vi "detection test.vi"() -> ()   [LabVIEW 2014]
uses:
  <vilib>/Math Plots/3D Math Plots/3D Ribbon/3D Ribbon XCtrl/3D Ribbon.xctl
  <vilib>/Math Plots/2D Math Plots/2D Compass/2D Compass XCtrl/2D Compass.xctl
  <vilib>/Math Plots/3D Math Plots/3D Ribbon/3D Ribbon Datatype/3D Ribbon Datatype.lvclass
  <vilib>/Math Plots/2D Math Plots/2D Compass/2D Compass Datatype/2D Compass Datatype.lvclass
panel:
  out "list":T1(array[cluster])
  in  "Take Reading":bool
  in  "Heading (deg)":dbl(knob)=90.0
  out "2D Compass":refnum<class "2D Plot Datatype.lvclass">[](xcontrol)
  out "Waveform Graph":dbl[][](graph)
  out "3D Ribbon":refnum<class "3D Plot Datatype.lvclass">[](xcontrol)
  in  "Stop":bool
  out "Zone":u8
  out "array":u8[](array[numeric])
  in  "Detectors":T2 {"Det 5" scale=0.0..255.0; "Det 4" scale=0.0..255.0; "Det 3" scale=0.0..255.0; "Det 2" scale=0.0..255.0; "Det 1" scale=0.0..255.0}
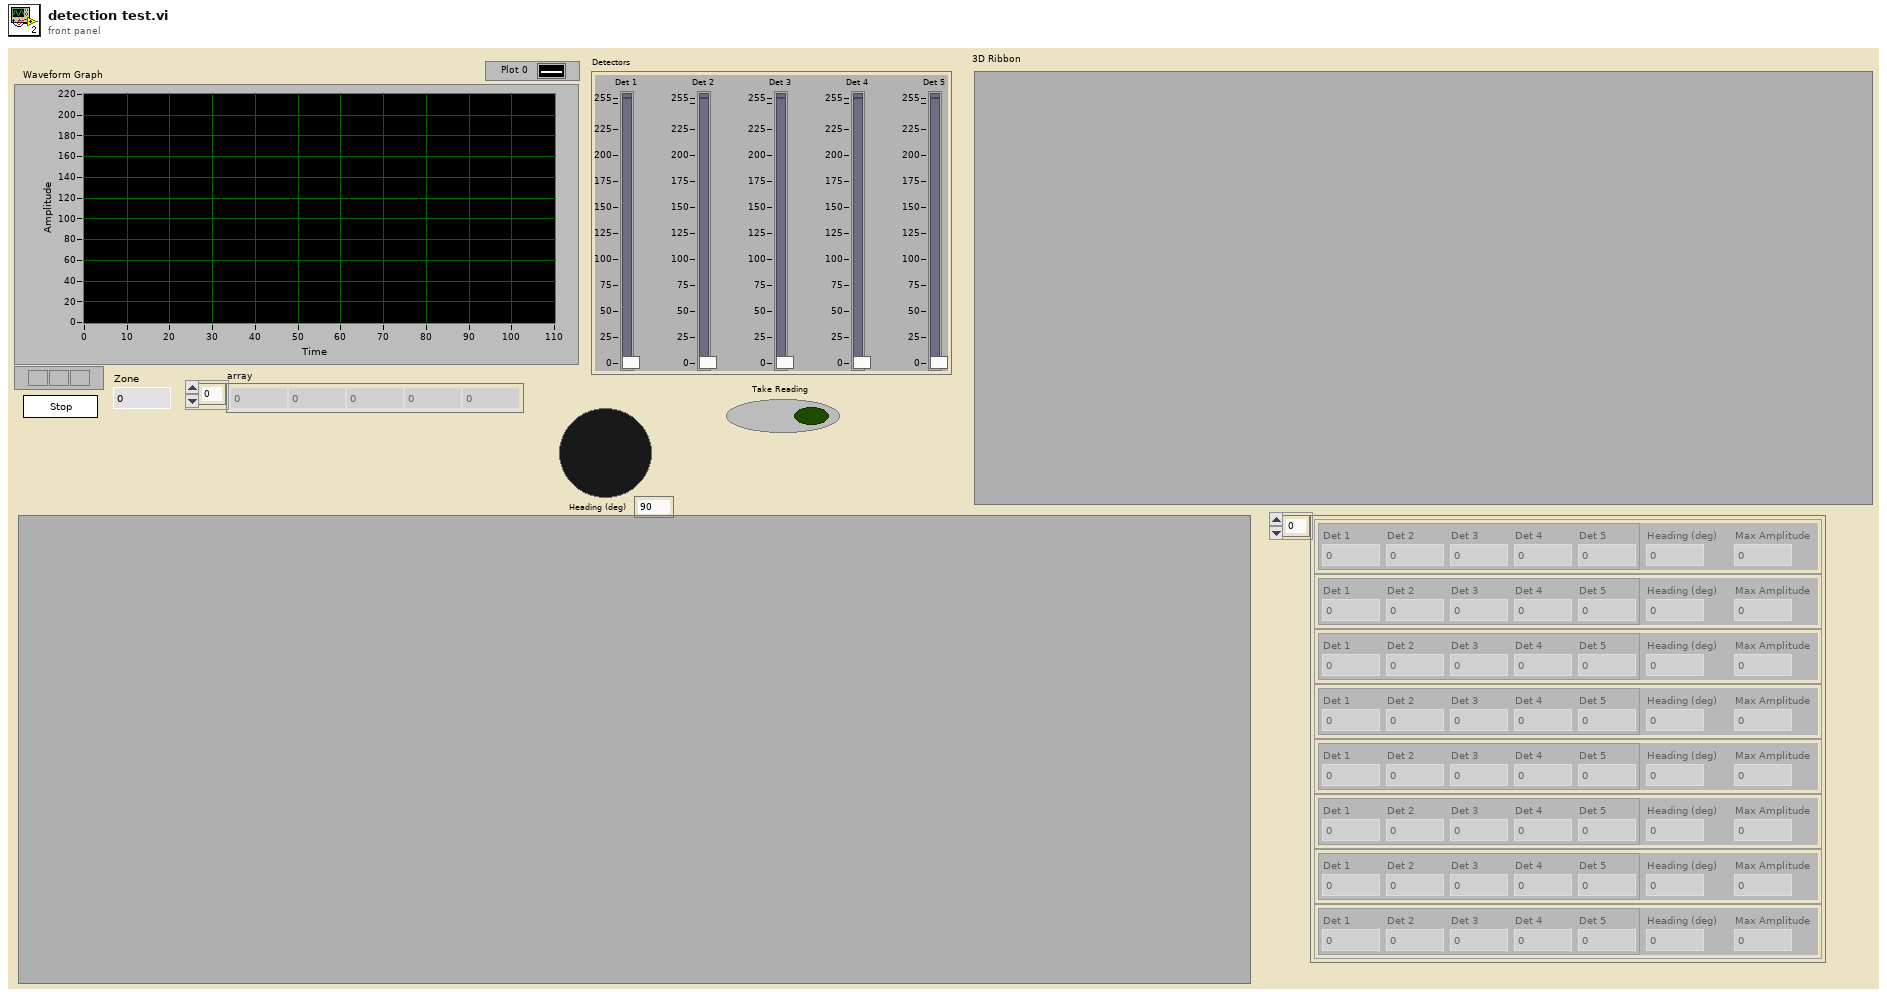
[diagram p1: front panel]
types:
  T1 = cluster{"Detectors":cluster{"Det 1":u8, "Det 2":u8, "Det 3":u8, "Det 4":u8, "Det 5":u8}, "Heading (deg)":dbl, "Max Amplitude":dbl}[]
  T2 = cluster{"Det 1":u8, "Det 2":u8, "Det 3":u8, "Det 4":u8, "Det 5":u8}
  T3 = cluster{"Detectors":cluster{"Det 1":u8, "Det 2":u8, "Det 3":u8, "Det 4":u8, "Det 5":u8}, "Heading (deg)":dbl, "Max Amplitude":dbl}
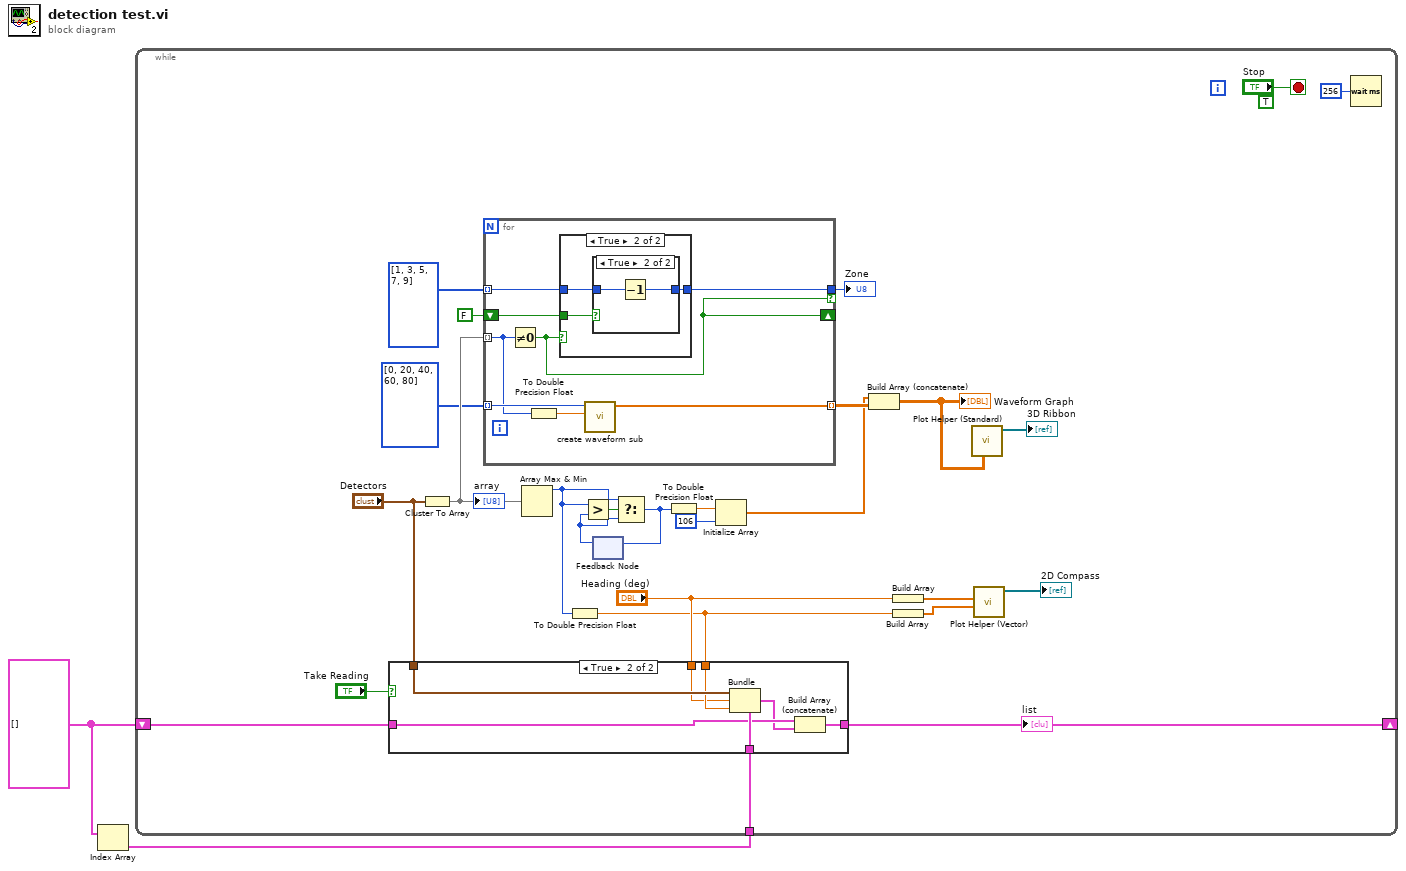
[diagram p0: block diagram]
diagram:
  w2 = T1 [] ("appended array")
  n1 = Index Array(array=w2) -> (element=w1:T3)  [unwired: 1 in]
  n2 = while {
    shift-right: [w10] -> _
    shift-left: w2 -> [w11]
    tunnel: w1 -> [w13]
    stop <- "Stop" stop-if-true
    (unwired) TRUE
    n3 = Cluster To Array(cluster="Detectors") -> (array=w26:u8[])
    "array" <- w26
    n4 = for {
      tunnel: w26 -> [w40] mode=indexing
      shift-right: [w42] -> _
      shift-left: FALSE -> [w45]
      tunnel: u8[] [1, 3, 5, 7, 9] ("array") -> [w44] mode=indexing
      tunnel: [w43] -> w27 if=w42
      tunnel: u8[] [0, 20, 40, 60, 80] ("array") -> [w41] mode=indexing
      tunnel: [w38] -> w20 mode=indexing
      n5 = Not Equal To 0?(x=w40) -> (x != 0?=w42:bool)
      n6 = To Double Precision Float(number=w40) -> (double precision float=w39:dbl)
      n7 = case shown="True" w42 {
        tunnel: w45 -> [_ w49]
        tunnel: w44 -> [w46 w48]
        tunnel: [w46 w47] -> w43
        frame False {
        }
        frame True {
          n8 = case shown="True" w49 {
            tunnel: [w50 w51] -> w47
            tunnel: w48 -> [w50 w52]
            frame False {
            }
            frame True {
              n9 = Decrement(x=w52) -> (x-1=w51:u8)
            }
          }
        }
      }
      n10 = call "create waveform sub.vi"("amplitude"=w39, "index"=w41) -> ("Array"=w38:dbl[])  [unwired: 9 in]
    }
    "Zone" <- w27
    n11 = Array Max & Min(array=w26) -> (max value=w4:u8)  [unwired: 3 out]
    n12 = To Double Precision Float(number=w4) -> (double precision float=w3:dbl)
    n13 = case shown="True" "Take Reading" {
      tunnel: "Detectors" -> [_ w37]
      tunnel: w3 -> [_ w36]
      tunnel: w13 -> [_ w35]
      tunnel: [w30 w34] -> w10
      tunnel: w11 -> [w30 w32]
      tunnel: "Heading (deg)" -> [_ w33]
      frame False {
      }
      frame True {
        n14 = Bundle(cluster=w35, "Detectors"=w37, "Heading (deg)"=w33, "Max Amplitude"=w36) -> (w31:T3)
        n15 = Build Array (concatenate)(w32, w31) -> (w34:T1)
      }
    }
    "list" <- w10
    n16 = feedback #1() -> (w24:u8)  [unwired: 1 in]
    n17 = Greater?(x=w4, y=w24) -> (0:w25:bool)
    n18 = Select(t=w4, s=w25, f=w24) -> (s? t:f=w23:u8)
    n19 = feedback-in #1(w23) -> ()
    n20 = To Double Precision Float(number=w23) -> (double precision float=w6:dbl)
    n21 = Initialize Array(w6, 106 ("dimension size")) -> (w19:dbl[])
    n22 = Build Array (concatenate)(w19, w20) -> (w15:dbl[][])
    "Waveform Graph" <- w15
    n23 = Build Array("Heading (deg)") -> (w8:dbl[])
    n24 = Build Array(w3) -> (w5:dbl[])
    n25 = call <vilib>:"Plot Helper (Standard).vi"("z matrix"=w15) -> ("3D Plot lvclass Array out"=→"3D Ribbon":refnum<class "3D Plot Datatype.lvclass">[])  [unwired: 9 in, 1 out]
    n26 = call <vilib>:"Plot Helper (Vector).vi"("radius vector"=w5, "theta vector"=w8) -> ("2D Plot Class Obj Array out"=→"2D Compass":refnum<class "2D Plot Datatype.lvclass">[])  [unwired: 8 in, 1 out]
    n27 = Wait (ms)(milliseconds to wait=u32 256) -> ()  [unwired: 1 out]
  }
